vi "Credito update.vi"(8 "error in (no error)":errorcluster, 10 "Credito":i32, 11 "Dinero in":refnum<class "Dinero.lvclass">) -> (0 "error out":errorcluster, 3 "Dinero out":refnum<class "Dinero.lvclass">)   [LabVIEW 2020, in "Dinero.lvlib" / "Dinero.lvclass"]
uses:
  Dinero.lvclass
  <vilib>/ActorFramework/Actor/Actor.lvclass
  User Interface Messages/Get dinero Msg/Get dinero Msg.lvclass
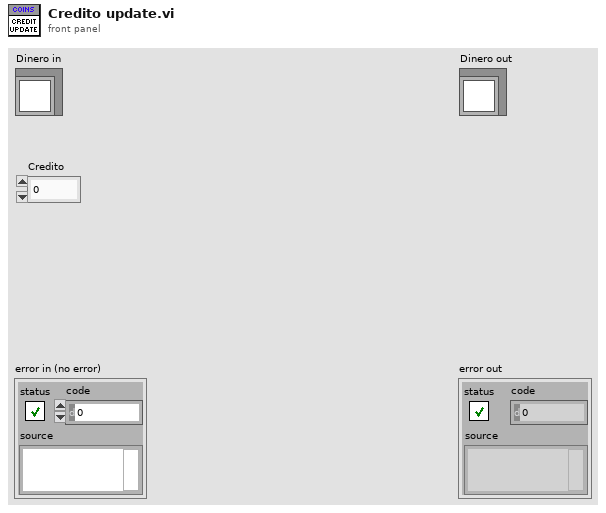
[diagram p1: front panel]
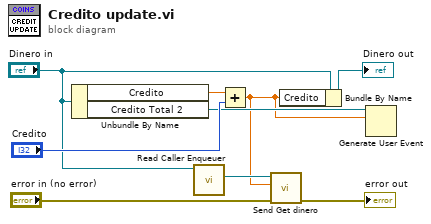
[diagram p0: block diagram]
diagram:
  n1 = Unbundle By Name("Dinero in") -> ("Credito"=w9:dbl, "Credito Total 2"=w6:refnum<user-event>)
  n2 = call <vilib>:"Read Caller Enqueuer.vi"("Actor"="Dinero in") -> ("Caller Enqueuer"=w4:refnum<class "Message Enqueuer.lvclass">)  [unwired: 10 in]
  n3 = Add(x=w9, y="Credito") -> (x+y=w3:dbl)
  n4 = call "Send Get dinero.vi"("error in (no error)"="error in (no error)", "Dinero"=w3, "Message Enqueuer"=w4) -> ("error out"=→"error out":errorcluster)  [unwired: 7 in, 1 out]
  n5 = Bundle By Name(cluster="Dinero in", "Credito"=w3) -> (→"Dinero out":refnum<class "Dinero.lvclass">)
  n6 = Generate User Event(user event=w6, event data cluster=w3) -> ()  [unwired: 2 in, 2 out]
